vi "4 channel fixed pixel clock resonance scanner acquisition (Host).vi"() -> ()   [LabVIEW 2012]
uses:
  <vilib>/rvi/interface/nirviOpenFPGA/nirviOpenFPGA.xnode
  <vilib>/rvi/interface/nirviMethod/nirviMethod.xnode
  <vilib>/rvi/interface/nirviReadWriteControl/nirviReadWriteControl.xnode
  <vilib>/rvi/errors/niLvFpgaMergeErrorWithErrorCode.vi
  <vilib>/rvi/interface/nirviCloseFPGA/nirviCloseFPGA.xnode
  <vilib>/DAQmx/create/channels.llb/DAQmx Create Channel (AO-Voltage-Basic).vi
  <vilib>/DAQmx/configure/timing.llb/DAQmx Timing (Sample Clock).vi
  <vilib>/DAQmx/write.llb/DAQmx Write (Analog 1D DBL 1Chan NSamp).vi
  <vilib>/DAQmx/configure/trigger.llb/DAQmx Start Trigger (Digital Edge).vi
  <vilib>/vision/NI_Vision_Development_Module.lvlib
  D/Dropbox/Scientifica SoftScan project/fpga testing/4 ch resonance scanner acquisition (FPGA) fixed pix clock.vi
  D/Dropbox/Scientifica SoftScan project/fpga testing/FPGA Bitfiles/4chresonancescan_PXIe-7962R_newLindsaymod4ch_VNbAuiLy9JE.lvbitx
  <vilib>/userdefined/High Color/nirio_resource_hc.ctl
panel:
  out "Timed Out":bool
  out "Numeric 2":i32
  out "Numeric":u32
  out "Array":i32[](array[numeric])
  out "ticks raw 4":i32[](graph) caption="interval between pixels in ticks"
  in  "data":dbl
  out "ticks raw 3":i32[](graph) caption="interval between pixels in ticks"
  in  "y-voltage":dbl=4.0
  in  "XOffset":i32
  out "error out":errorcluster
  in  "stop":bool
  out "Image":T1(plugin-control)
  in  "Requested Depth":u32=100000000
  out "ticks raw 2":i32[][](graph) caption="ticks raw"
  in  "lines at once":i32=100
  out "Actual Depth 3":u32
  out "Actual Depth":u32
  out "ch1":i32[][](graph)
  in  "Start Delay (Ticks)":i16
  in  "RIO Device":T2="RIO0"
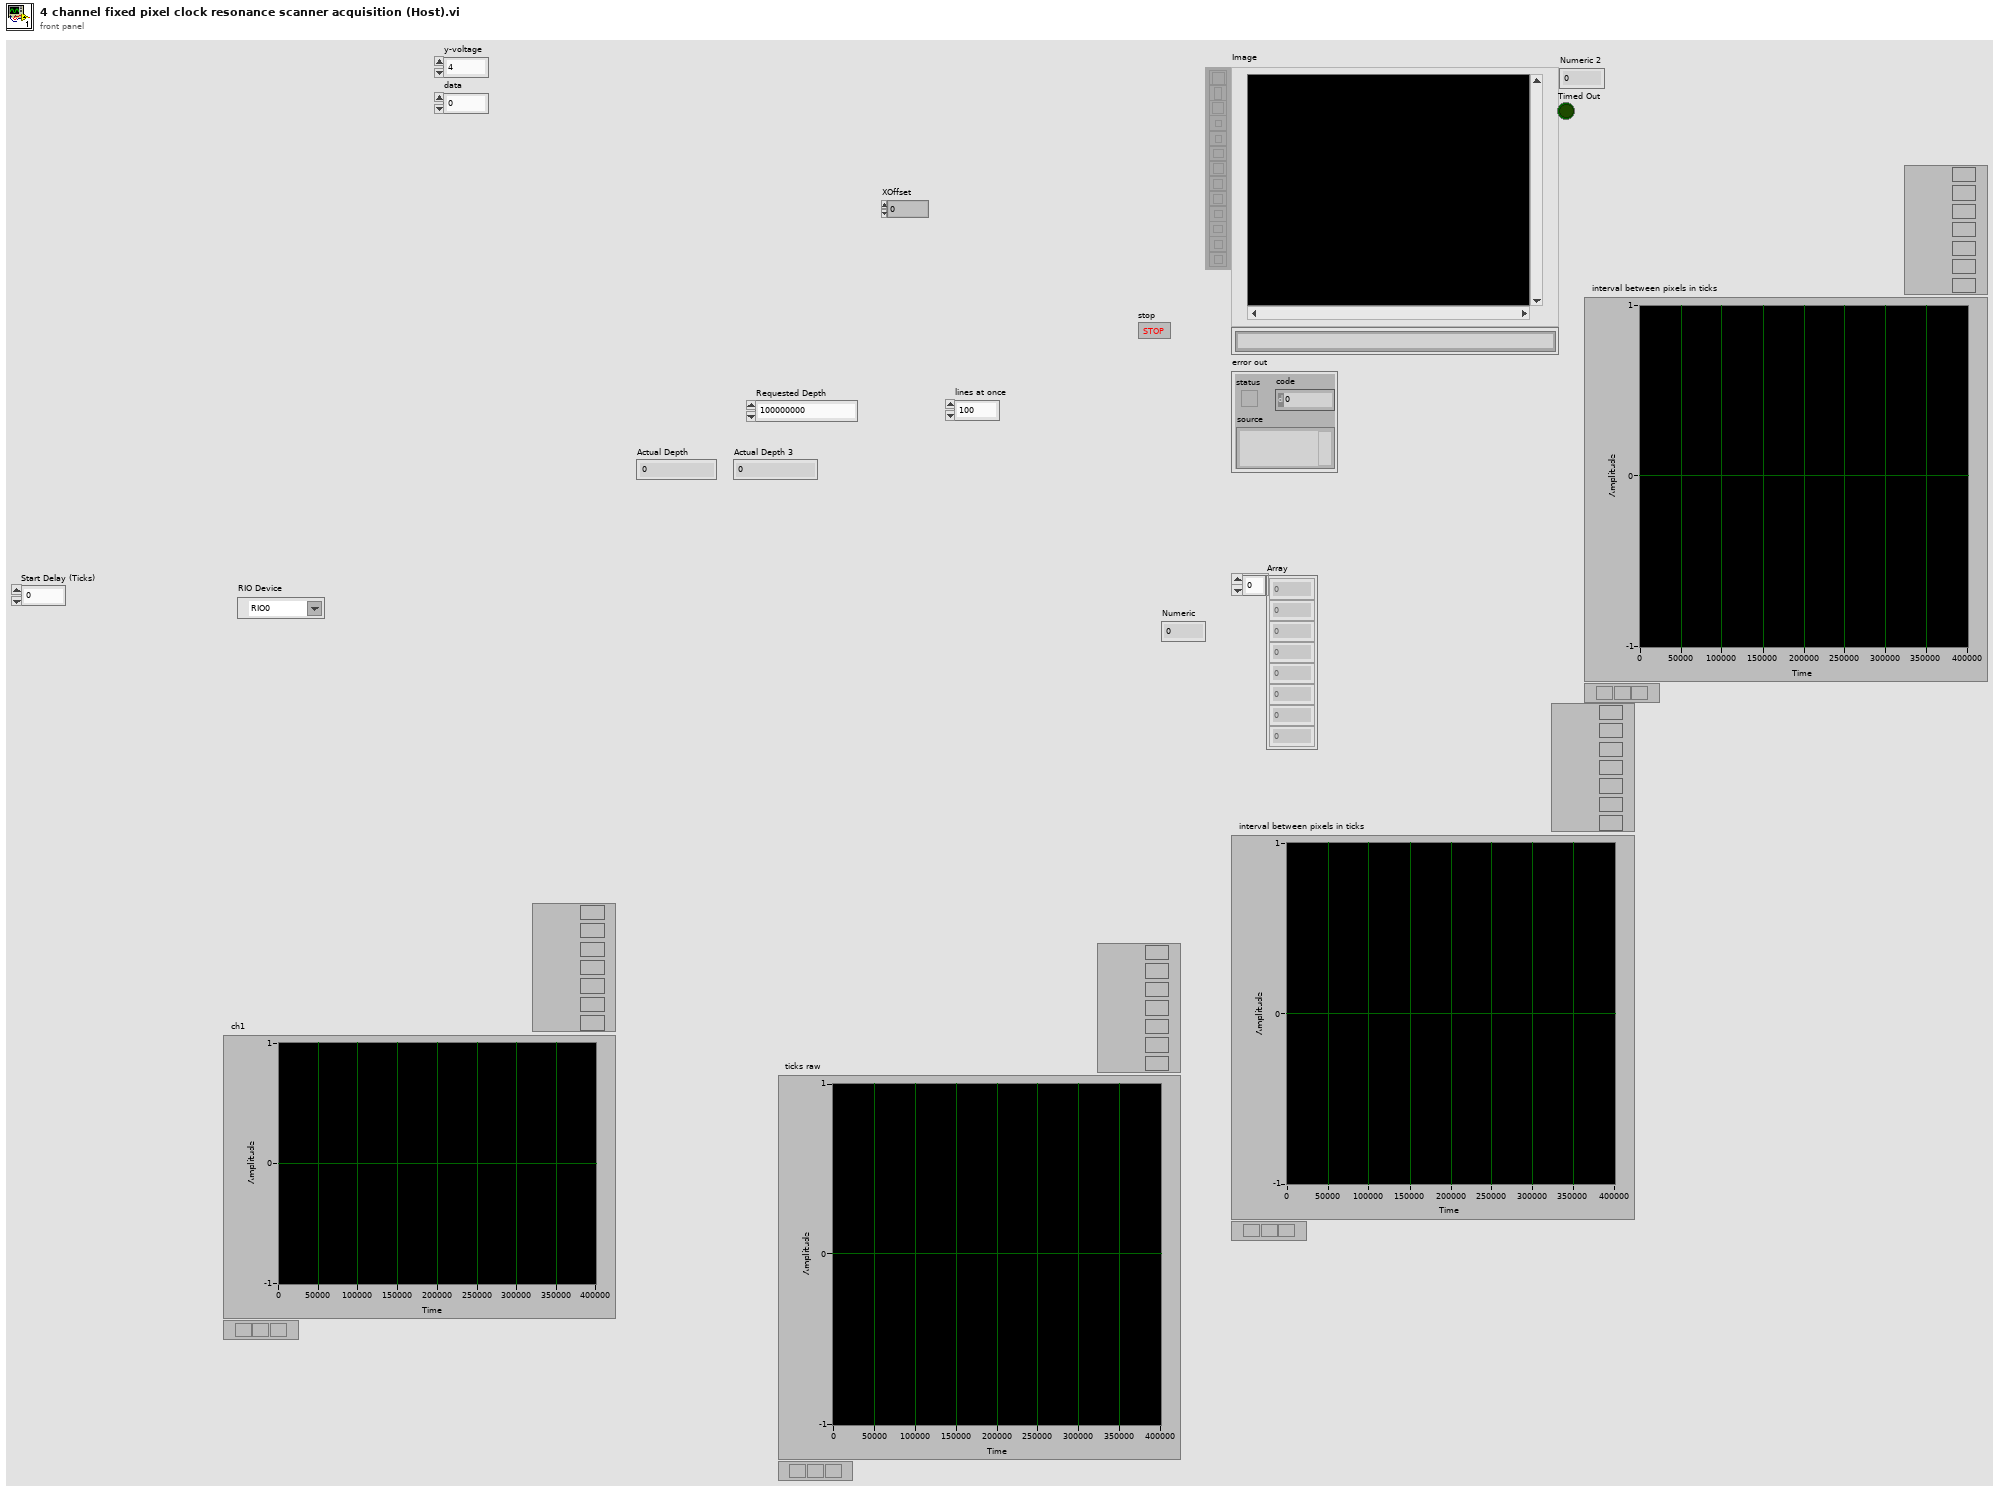
[diagram p1: front panel]
types:
  T1 = typedef "IMAQ Image.ctl" = refnum<image>
  T2 = typedef "nirio_resource_hc.ctl" = tag
  T3 = typedef "Image Type" = u32
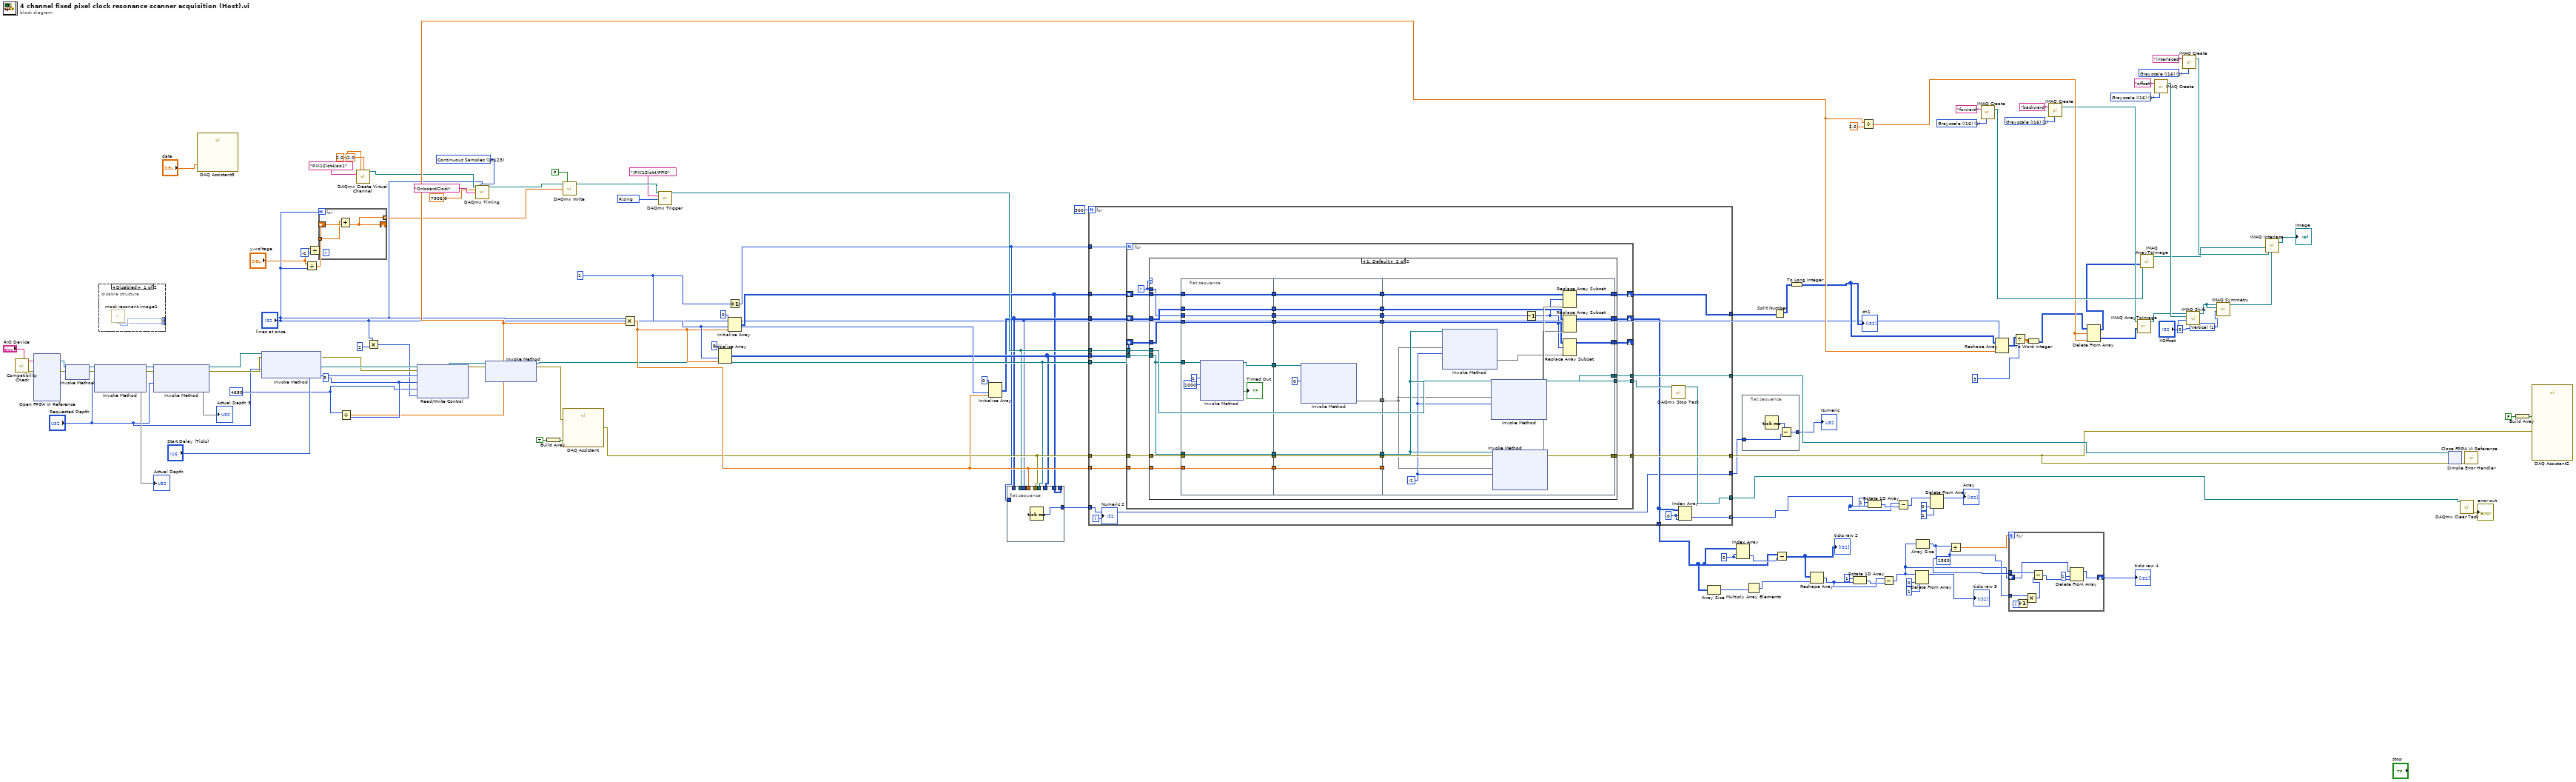
[diagram p0: block diagram]
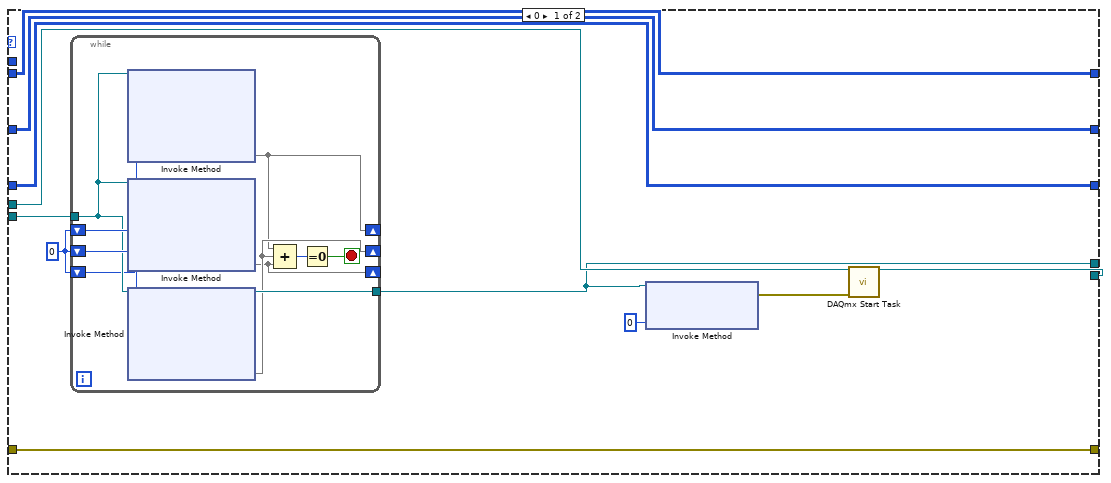
[diagram p2: hidden frame]
diagram:
  w26 = 1560 ("y")
  w48 = 10123 items=["Finite Samples"=10178, "Continuous Samples"=10123, "Hardware Timed Single Point"=12522] ("sample mode")
  w60 = u32 1 items=["Horizontal", "Vertical", "Central", "1st Diagonal", "2nd Diagonal"] ("Type of Symmetry")
  w76 = 0 ("disabled index (col)")
  w82 = 3 ("dwell time in ticks")
  w81 = i16 4680 ("samples per period")
  w87 = T3 1 items=["Grayscale (U8)", "Grayscale (I16)", "Grayscale (SGL)", "Complex (CSG)", "RGB (U32)", "HSL (U32)", "RGB (U64)", "Grayscale (U16)"] ("Image Type")
  w91 = T3 1 items=["Grayscale (U8)", "Grayscale (I16)", "Grayscale (SGL)", "Complex (CSG)", "RGB (U32)", "HSL (U32)", "RGB (U64)", "Grayscale (U16)"] ("Image Type")
  w93 = T3 1 items=["Grayscale (U8)", "Grayscale (I16)", "Grayscale (SGL)", "Complex (CSG)", "RGB (U32)", "HSL (U32)", "RGB (U64)", "Grayscale (U16)"] ("Image Type")
  w97 = 10280 items=["Rising"=10280, "Falling"=10171] ("edge")
  w104 = T3 1 items=["Grayscale (U8)", "Grayscale (I16)", "Grayscale (SGL)", "Complex (CSG)", "RGB (U32)", "HSL (U32)", "RGB (U64)", "Grayscale (U16)"] ("Image Type")
  w44 = 1 ("Numeric")
  n1 = call "Compatibility Check.vi"() -> ("error out"=w123:errorcluster)  [unwired: 2 in, 9 out]
  n2 = xnode "Open FPGA VI Reference"("error in"=w123, "resource name"="RIO Device") -> ("FPGA VI Reference Out"=w120:refnum<k20>, "error out"=w121:errorcluster)
  n3 = xnode "Invoke Method"("FPGA VI Reference In"=w120, "error in"=w121) -> ("FPGA VI Reference Out"=w118:refnum<k20>, "error out"=w85:errorcluster)
  n4 = xnode "Invoke Method"("FPGA VI Reference In"=w118, "error in"=w85, "Requested Depth"="Requested Depth") -> ("FPGA VI Reference Out"=w112:refnum<k20>, "error out"=w84:errorcluster, "Actual Depth"=→"Actual Depth")
  n5 = disable-structure shown="Disabled" {
    disable-tunnel: [w125 _] -> _
    disable-tunnel: [w124 _] -> _
    frame Disabled {
      n6 = call "mock resonant image1.vi"() -> ("samples per period (fix pix clock)"=w125:i32, "fixed dwell time"=w124:i32)  [unwired: 7 in, 3 out]
    }
    frame Enabled {
    }
  }
  n7 = xnode "Invoke Method"("FPGA VI Reference In"=w112, "error in"=w84, "Requested Depth"="Requested Depth") -> ("FPGA VI Reference Out"=w35:refnum<k20>, "error out"=w34:errorcluster, "Actual Depth"=→"Actual Depth 3")
  n8 = call "DAQ Assistant3"("data"="data") -> ()  [unwired: 17 in, 2 out]
  n9 = xnode "Invoke Method"("FPGA VI Reference In"=w35, "error in"=w34, "Requested Depth"="Requested Depth") -> ("FPGA VI Reference Out"=w33:refnum<k20>, "error out"=w32:errorcluster)  [unwired: 1 out]
  n10 = Divide(x="y-voltage", y="lines at once") -> (x/y=w57:dbl)
  n11 = Divide(x="y-voltage", y=-2) -> (x/y=w55:dbl)
  n12 = for {
    N: "lines at once" -> [_]
    tunnel: w57 -> [w127]
    shift-right: [w126] -> _
    shift-left: w55 -> [w128]
    tunnel: [w126] -> w52 mode=indexing
    n13 = Add(x=w127, y=w128) -> (x+y=w126:dbl)
  }
  n14 = Divide(x=w81, y=w82) -> (x/y=w80:dbl)
  n15 = call-poly <vilib>:"DAQmx Create Virtual Channel.vi"("maximum value"=2.0, "minimum value"=-2.0, "physical channels"=tag "PXI1Slot4/ao1") -> ("task out"=w59:refnum<k21>)  [unwired: 11 in, 1 out]
  n16 = Multiply(x="lines at once", y=2) -> (x*y=w2:i32)
  n17 = xnode "Read/Write Control"("FPGA VI Reference In"=w33, "error in"=w32, "Start Delay (Ticks)"="Start Delay (Ticks)", "dwell time in ticks"=w82, "samples per period"=w81, "lines at once"=w2) -> ("FPGA VI Reference Out"=w117:refnum<k20>, "error out"=w83:errorcluster)
  n18 = call-poly <vilib>:"DAQmx Timing.vi"("task/channels in"=w59, "sample mode"=w48, "samples per channel"="lines at once", "rate"=7906.0, "source"=tag "OnboardClock") -> ("task out"=w54:refnum<k21>)  [unwired: 9 in, 1 out]
  n19 = xnode "Invoke Method"("FPGA VI Reference In"=w117, "error in"=w83) -> ("FPGA VI Reference Out"=w12:refnum<k20>, "error out"=w79:errorcluster)  [unwired: 1 in]
  n20 = Build Array(TRUE) -> (w110:bool[])
  n21 = call-poly <vilib>:"DAQmx Write.vi"("task/channels in"=w54, "auto start"=FALSE, "data"=w52) -> ("task out"=w99:refnum<k21>)  [unwired: 10 in, 2 out]
  n22 = call "DAQ Assistant"("data"=w110, "error in"=w79) -> ("error out"=w13:errorcluster)  [unwired: 16 in, 1 out]
  n23 = Multiply(x="lines at once", y=w80) -> (x*y=w14:dbl)
  n24 = call-poly <vilib>:"DAQmx Trigger.vi"("task/channels in"=w99, "source"=tag "/PXI1Slot4/PFI0", "edge"=w97) -> ("task out"=w10:refnum<k21>)  [unwired: 11 in, 1 out]
  n25 = Initialize Array(u64 0 ("element"), w44, w14) -> (w11:u64[][])
  n26 = Initialize Array(u64 0 ("element"), w44, w14) -> (w8:u64[][])
  n27 = Increment(x=w44) -> (x+1=w7:i32)
  n28 = Initialize Array(0 ("element"), w44, w14) -> (w9:i32[][])
  n29 = flat-sequence {
    tunnel: w14 -> [_]
    tunnel: w13 -> [_]
    tunnel: w12 -> [_]
    tunnel: w11 -> [_]
    tunnel: w10 -> [_]
    tunnel: "lines at once" -> [_]
    tunnel: w9 -> [_]
    tunnel: [w130] -> _
    tunnel: w8 -> [w130]
    tunnel: w7 -> [_]
    tunnel: [w129] -> w6
    frame #0 {
      n30 = Tick Count (ms)() -> (millisecond timer value=w129:u32)
    }
  }
  n31 = for {
    N: 300 -> [_]
    tunnel: w7 -> [w148]
    tunnel: w8 -> [w147]
    tunnel: w9 -> [w146]
    tunnel: [w145] -> w108
    tunnel: [w144] -> w105
    tunnel: [w143] -> w101
    tunnel: [w142] -> w77
    tunnel: w12 -> [w140]
    tunnel: w13 -> [w139]
    tunnel: w10 -> [w138]
    tunnel: w14 -> [w137]
    tunnel: w11 -> [w136]
    tunnel: [w135] -> w43
    tunnel: [w133] -> w16 mode=indexing
    tunnel: w6 -> [w132]
    tunnel: [w132] -> w5
    i -> [w131]
    w134 = 0 ("index (row)")
    n32 = for {
      N: w148 -> [_]
      tunnel: w140 -> [w160]
      tunnel: [w162] -> w144
      tunnel: w137 -> [w161]
      shift-right: [w157] -> w142
      shift-left: w147 -> [w158]
      shift-right: [w156] -> w135
      shift-left: w146 -> [w159]
      tunnel: [w155] -> w145
      tunnel: w138 -> [w154]
      tunnel: [w153] -> w141
      tunnel: w139 -> [w149]
      shift-right: [w150] -> _
      shift-left: w136 -> [w151]
      i -> [w152]
      n33 = case shown="1, Default" w152 {
        tunnel: [w167 w212] -> w162
        tunnel: w161 -> [_ w201]
        tunnel: w160 -> [w172 w200]
        tunnel: w159 -> [w171 w211]
        tunnel: w158 -> [w173 w210]
        tunnel: [w173 w209] -> w157
        tunnel: [w171 w208] -> w156
        tunnel: w152 -> [_ w206]
        tunnel: [w164 w207] -> w155
        tunnel: w154 -> [w170 w205]
        tunnel: [w169 w205] -> w153
        tunnel: w151 -> [w166 w204]
        tunnel: [w166 w203] -> w150
        tunnel: w149 -> [w167 w202]
        frame 0 {
          w168 = u32 0 ("Elements Remaining")
          n34 = while {
            tunnel: w172 -> [w178]
            tunnel: [w179] -> w164
            shift-right: [w174] -> _
            shift-left: w168 -> [w182]
            shift-right: [w176] -> _
            shift-left: w168 -> [w183]
            shift-right: [w175] -> _
            shift-left: w168 -> [w177]
            stop <- w180 stop-if-true
            n35 = xnode "Invoke Method"("FPGA VI Reference In"=w178, "Number of Elements"=w182) -> ("Elements Remaining"=w174)  [unwired: 2 in, 3 out]
            n36 = xnode "Invoke Method"("FPGA VI Reference In"=w178, "Number of Elements"=w177) -> ("Elements Remaining"=w175)  [unwired: 2 in, 3 out]
            n37 = xnode "Invoke Method"("FPGA VI Reference In"=w178, "Number of Elements"=w183) -> ("FPGA VI Reference Out"=w179:refnum<k20>, "Elements Remaining"=w176)  [unwired: 2 in, 2 out]
            n38 = Compound Arithmetic op=unknown(w174, w176, w175) -> (w181:i32)
            n39 = Equal To 0?(x=w181) -> (x = 0?=w180:bool)
          }
          n40 = xnode "Invoke Method"("FPGA VI Reference In"=w164, "IRQ Number(s)"=0) -> ("error out"=w163:errorcluster)  [unwired: 1 in, 1 out]
          n41 = call <vilib>:"DAQmx Start Task.vi"("task/channels in"=w170, "error in"=w163) -> ("task out"=w169:refnum<k21>)  [unwired: 12 in, 1 out]
        }
        frame 1, Default {
          n42 = flat-sequence {
            tunnel: w201 -> [w218]
            tunnel: w200 -> [w219]
            tunnel: w202 -> [w220]
            tunnel: w204 -> [w221]
            tunnel: w206 -> [w222]
            tunnel: w210 -> [w223]
            tunnel: w211 -> [w224]
            tunnel: [w224] -> w199
            tunnel: [w223] -> w197
            tunnel: [w222] -> w195
            tunnel: [w221] -> w193
            tunnel: [w220] -> w191
            tunnel: [w219] -> w189
            tunnel: [w218] -> w187
            tunnel: w200 -> [w216]
            tunnel: [w213] -> w185
            tunnel: w199 -> [w234]
            tunnel: [w234] -> w198
            tunnel: w197 -> [w233]
            tunnel: [w233] -> w196
            tunnel: w195 -> [w232]
            tunnel: [w232] -> w194
            tunnel: w193 -> [w231]
            tunnel: [w231] -> w192
            tunnel: w191 -> [w230]
            tunnel: [w230] -> w190
            tunnel: w189 -> [w229]
            tunnel: [w229] -> w188
            tunnel: w187 -> [w228]
            tunnel: [w228] -> w186
            tunnel: w185 -> [w226]
            tunnel: [w225] -> w184
            tunnel: [w250] -> w212
            tunnel: [w246] -> w209
            tunnel: [w245] -> w208
            tunnel: [w244] -> w207
            tunnel: [w239] -> w203
            tunnel: w198 -> [w249]
            tunnel: w196 -> [w248]
            tunnel: w194 -> [w243]
            tunnel: w192 -> [w242]
            tunnel: w190 -> [w238]
            tunnel: w188 -> [w237]
            tunnel: w186 -> [_]
            tunnel: w184 -> [w235]
            frame #0 {
              n43 = xnode "Invoke Method"("FPGA VI Reference In"=w216, "IRQ Number(s)"=1, "Timeout (ms)"=1000) -> ("FPGA VI Reference Out"=w213:refnum<k20>, "Timed Out"=→"Timed Out")  [unwired: 1 in, 2 out]
            }
            frame #1 {
              n44 = xnode "Invoke Method"("FPGA VI Reference In"=w226, "Number of Elements"=u32 0) -> ("Elements Remaining"=w225)  [unwired: 2 in, 3 out]
            }
            frame #2 {
              w236 = -1 ("Timeout (ms)")
              n45 = xnode "Invoke Method"("FPGA VI Reference In"=w237, "Number of Elements"=w235, "Timeout (ms)"=w236) -> ("Data"=w240:void[])  [unwired: 1 in, 3 out]
              n46 = xnode "Invoke Method"("FPGA VI Reference In"=w237, "Number of Elements"=w235, "Timeout (ms)"=w236) -> ("FPGA VI Reference Out"=w244:refnum<k20>, "Data"=w247:void[])  [unwired: 1 in, 2 out]
              n47 = xnode "Invoke Method"("FPGA VI Reference In"=w237, "error in"=w238, "Number of Elements"=w235, "Timeout (ms)"=w236) -> ("error out"=w250:errorcluster, "Data"=w251:void[])  [unwired: 2 out]
              n48 = Decrement(x=w243) -> (x-1=w241:i32)
              n49 = Replace Array Subset(array=w248, new element=w251, index (row)=w241) -> (w246:u64[][])  [unwired: 1 in]
              n50 = Replace Array Subset(array=w249, new element=w247, index (row)=w241) -> (w245:i32[][])  [unwired: 1 in]
              n51 = Replace Array Subset(array=w242, new element=w240, index (row)=w241) -> (w239:u64[][])  [unwired: 1 in]
            }
          }
        }
      }
    }
    n52 = call <vilib>:"DAQmx Stop Task.vi"("task/channels in"=w141) -> ("task out"=w143:refnum<k21>)  [unwired: 13 in, 1 out]
    n53 = Index Array(array=w135, index (row)=w134, index (col)=w134) -> (element=w133:i32)
    "Numeric 2" <- w131
  }
  n54 = Array Size(array=w43) -> (size(s)=w41:i32[])
  n55 = Index Array(array=w43, index (row)=w76, index (col)=w76) -> (element=w75:i32)
  n56 = flat-sequence {
    tunnel: w5 -> [w253]
    tunnel: [w252] -> w4
    frame #0 {
      n57 = Tick Count (ms)() -> (millisecond timer value=w254:u32)
      n58 = Subtract(x=w254, y=w253) -> (x-y=w252:u32)
    }
  }
  n59 = Multiply Array Elements(1:w41) -> (0:w40:i32)
  n60 = Split Number(x=w77) -> (hi(x)=w78:u32[][])  [unwired: 1 out]
  n61 = Subtract(x=w43, y=w75) -> (x-y=w42:i32[][])
  "ticks raw 2" <- w42
  n62 = To Long Integer(number=w78) -> (32bit integer=w74:i32[][])
  "ch1" <- w74
  n63 = Reshape Array(w42, w40) -> (w38:i32[])
  n64 = Rotate 1D Array(1:w38, 2:1 ("n")) -> (0:w37:i32[])
  n65 = Divide(x=w80, y=2.0) -> (x/y=w95:dbl)
  n66 = Rotate 1D Array(1:w16, 2:1 ("n")) -> (0:w18:i32[])
  n67 = Subtract(x=w38, y=w37) -> (x-y=w24:i32[])
  n68 = Subtract(x=w16, y=w18) -> (x-y=w21:i32[])
  n69 = Delete From Array(array=w24, length=1, index=0) -> (array with subset deleted=→"ticks raw 3":i32[])  [unwired: 1 out]
  n70 = Array Size(array=w24) -> (size(s)=w27:i32)
  n71 = Delete From Array(array=w21, length=1, index=0) -> (array with subset deleted=→"Array":i32[])  [unwired: 1 out]
  n72 = Divide(x=w27, y=w26) -> (x/y=w28:dbl)
  n73 = call "IMAQ Create"("Image Name"="forward", "Image Type"=w104) -> ("New Image"=w102:T1)  [unwired: 3 in, 1 out]
  n74 = Reshape Array(w74, "lines at once", w80) -> (w72:i32[][])
  n75 = for {
    N: w28 -> [_]
    tunnel: w27 -> [w263]
    tunnel: w26 -> [w260]
    shift-right: [w255] -> w23
    shift-left: w24 -> [w256]
    i -> [w262]
    n76 = Increment(x=w262) -> (x+1=w261:i32)
    n77 = Multiply(x=w260, y=w261) -> (x*y=w259:i32)
    n78 = Subtract(x=w263, y=w259) -> (x-y=w258:i32)
    n79 = Delete From Array(array=w256, length=1, index=w258) -> (array with subset deleted=w255:i32[])  [unwired: 1 out]
  }
  "ticks raw 4" <- w23
  n80 = Divide(x=w72, y=3 ("element")) -> (x/y=w73:dbl[][])
  n81 = To Word Integer(number=w73) -> (16bit integer=w70:i16[][])
  n82 = call "IMAQ Create"("Image Name"="backward", "Image Type"=w93) -> ("New Image"=w92:T1)  [unwired: 3 in, 1 out]
  n83 = Delete From Array(array=w70, length=w95, index (col)=w95) -> (deleted portion=w68:i16[][], array with subset deleted=w69:i16[][])  [unwired: 1 in]
  n84 = call "IMAQ ArrayToImage"("Image Pixels (I16)"=w68, "Image"=w92) -> ("Image Out"=w67:T1)  [unwired: 8 in, 1 out]
  n85 = call "IMAQ ArrayToImage"("Image Pixels (I16)"=w69, "Image"=w102) -> ("Image Out"=w63:T1)  [unwired: 8 in, 1 out]
  n86 = call "IMAQ Create"("Image Name"="offset", "Image Type"=w91) -> ("New Image"=w89:T1)  [unwired: 3 in, 1 out]
  n87 = call "IMAQ Create"("Image Name"="interlaced", "Image Type"=w87) -> ("New Image"=w86:T1)  [unwired: 3 in, 1 out]
  n88 = call "IMAQ Shift"("YOffset"=0, "XOffset"="XOffset", "Image Dst"=w89, "Image Src"=w67) -> ("Image Dst Out"=w62:T1)  [unwired: 6 in, 1 out]
  n89 = call "IMAQ Symmetry"("Type of Symmetry"=w60, "Image Dst"=w62, "Image Src"=w62) -> ("Image Dst Out"=w61:T1)  [unwired: 2 in, 1 out]
  n90 = call "IMAQ Interlace"("Image Even"=w63, "Image Odd"=w61, "Image Frame"=w86) -> ("Image Frame Out"=→"Image":T1)  [unwired: 2 in, 3 out]
  n91 = xnode "Close FPGA VI Reference"("FPGA VI Reference In"=w108, "error in"=w105) -> ("error out"=w109:errorcluster)
  n92 = call <vilib>:"DAQmx Clear Task.vi"("task in"=w101) -> ("error out"=→"error out":errorcluster)  [unwired: 14 in]
  n93 = call <vilib>:"Simple Error Handler.vi"("error in (no error)"=w109) -> ()  [unwired: 1 in, 8 out]
  n94 = Build Array(FALSE) -> (w106:bool[])
  n95 = call "DAQ Assistant2"("data"=w106, "error in"=w105) -> ()  [unwired: 16 in, 2 out]
  "Numeric" <- w4
